vi "Init Stream.vi"(0 "Target IPAddress":string) -> ()   [LabVIEW 2015]
panel:
  out "Tab Control":enum32{"ON", "Off"}(tab)
  in  "Start":bool
  # "Start"
  # "Hi!\nThere are a few settings you will have to configure for the robot to run..."
  # "Please wait. Loading..."
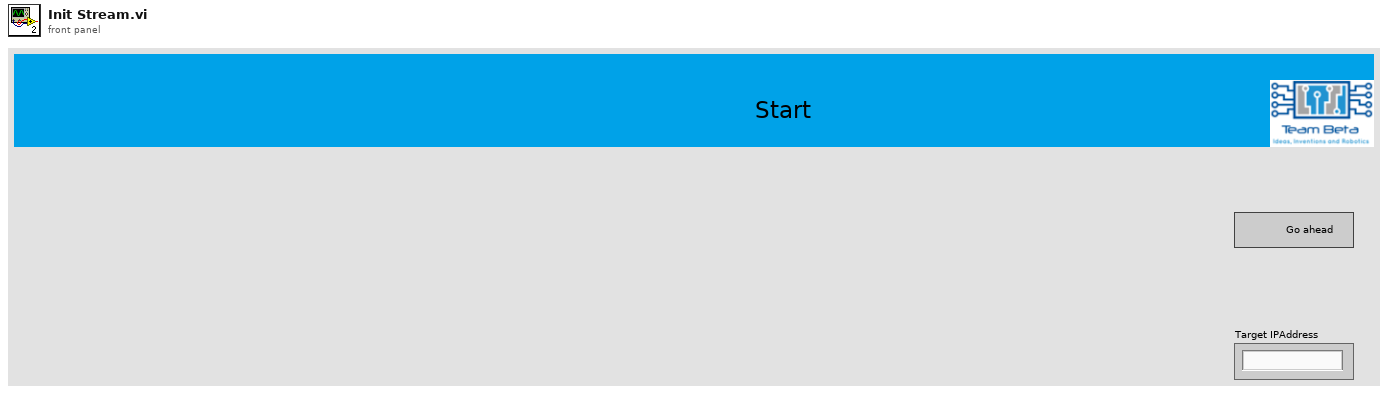
[diagram p1: front panel]
types:
  T1 = typedef "MODE.ctl" = enum8{"Protected Manaul", "Automatic", "Manaul"}
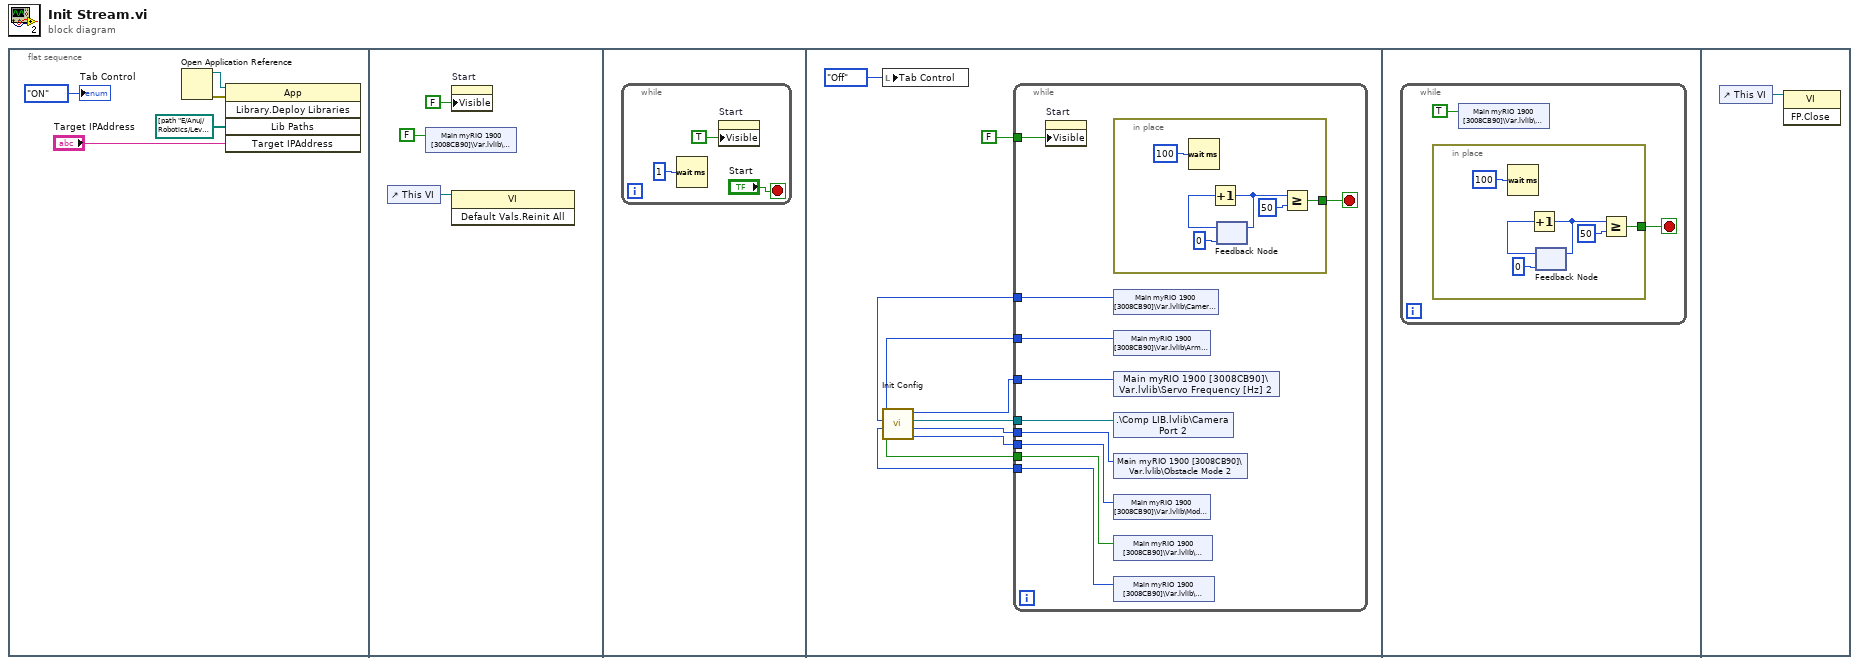
[diagram p0: block diagram]
diagram:
  n1 = flat-sequence {
    frame #0 {
      n2 = Open Application Reference() -> (0:w4:errorcluster, 3:w3:refnum<vi>)  [unwired: 4 in]
      n3 = invoke class="App" method="Library.Deploy Libraries"(reference=w3, error in=w4, "Lib Paths"=path[] [path "E:/Anuj/Robotics/Level 3/LabVIEW/Main VIs/LV15/PDMS/Real Time/Var.lvlib"] ("Library Paths"), "Target IPAddress"="Target IPAddress") -> ()  [unwired: 1 in, 5 out]
      "Tab Control" <- enum32{"ON", "Off"}."ON" ("Tab Control")
    }
    frame #1 {
      n4 = control-ref of="This VI"() -> (w8:refnum<vi>)
      n5 = shared-variable "Main myRIO 1900 [3008CB90]\\Var.lvlib\\Start-init"(FALSE ("Stop-init")) -> ()  [unwired: 1 in, 1 out]
      n6 = property on="Start" class="Bool"("Visible"=FALSE) -> ()  [unwired: 2 in, 2 out]
      n7 = invoke class="VI" method="Default Vals.Reinit All"(reference=w8) -> ()  [unwired: 2 in, 3 out]
    }
    frame #2 {
      n8 = while {
        stop <- "Start" stop-if-true
        n9 = Wait (ms)(milliseconds to wait=u32 1 ("millisecond timer value")) -> ()  [unwired: 1 out]
        n10 = property on="Start" class="Bool"("Visible"=TRUE) -> ()  [unwired: 2 in, 2 out]
      }
    }
    frame #3 {
      n11 = local write "Tab Control"(enum32{"ON", "Off"}."Off" ("Tab Control")) -> ()
      n12 = call "Init Config.vi"() -> ("Mode out"=w18:T1, "Obstacle Mode 2"=w19:u16, "Camera Port 2"=w15:refnum<k21>, "Servo Frequency [Hz] 2"=w20:u32, "Canceled?"=w17:bool, "Obstacle??"=w14:enum32{"Radio Selection 1", "Radio Selection 2"}, "Camera YN"=w13:enum32{"Radio Selection 1", "Radio Selection 2"}, "Arm Type"=w16:enum32{"RS1", "RS2"})  [unwired: 4 in]
      n13 = while {
        tunnel: FALSE ("Visible") -> [w30]
        tunnel: w20 -> [w29]
        tunnel: w19 -> [w28]
        tunnel: w18 -> [w27]
        tunnel: w17 -> [w26]
        tunnel: w16 -> [w25]
        tunnel: w15 -> [w24]
        tunnel: w14 -> [w23]
        tunnel: w13 -> [w22]
        stop <- w31 stop-if-true
        n14 = property on="Start" class="Bool"("Visible"=w30) -> ()  [unwired: 2 in, 2 out]
        n15 = in-place {
          in-place-border: [w32] -> w31
          n16 = Wait (ms)(milliseconds to wait=u32 100 ("millisecond timer value")) -> ()  [unwired: 1 out]
          n17 = feedback #1(u16 0) -> (w37:u16)
          n18 = Increment(x=w37) -> (x+1=w35:u16)
          n19 = feedback-in #1(w35) -> ()
          n20 = Greater Or Equal?(x=w35, y=u16 50) -> (x >= y?=w32:bool)
        }
        n21 = shared-variable "Main myRIO 1900 [3008CB90]\\Var.lvlib\\Camera YN"(w22) -> ()  [unwired: 1 in, 1 out]
        n22 = shared-variable "Main myRIO 1900 [3008CB90]\\Var.lvlib\\Arm Type"(w25) -> ()  [unwired: 1 in, 1 out]
        n23 = shared-variable "Main myRIO 1900 [3008CB90]\\Var.lvlib\\Servo Frequency [Hz] 2"(w29) -> ()  [unwired: 1 in, 1 out]
        n24 = shared-variable ".\\Comp LIB.lvlib\\Camera Port 2"(w24) -> ()  [unwired: 1 in, 1 out]
        n25 = shared-variable "Main myRIO 1900 [3008CB90]\\Var.lvlib\\Obstacle Mode 2"(w28) -> ()  [unwired: 1 in, 1 out]
        n26 = shared-variable "Main myRIO 1900 [3008CB90]\\Var.lvlib\\Mode out"(w27) -> ()  [unwired: 1 in, 1 out]
        n27 = shared-variable "Main myRIO 1900 [3008CB90]\\Var.lvlib\\Canceled?"(w26) -> ()  [unwired: 1 in, 1 out]
        n28 = shared-variable "Main myRIO 1900 [3008CB90]\\Var.lvlib\\Obstacle??"(w23) -> ()  [unwired: 1 in, 1 out]
      }
    }
    frame #4 {
      n29 = while {
        stop <- w38 stop-if-true
        n30 = in-place {
          in-place-border: [w40] -> w38
          n31 = Wait (ms)(milliseconds to wait=u32 100 ("millisecond timer value")) -> ()  [unwired: 1 out]
          n32 = feedback #2(u16 0) -> (w45:u16)
          n33 = Increment(x=w45) -> (x+1=w43:u16)
          n34 = feedback-in #2(w43) -> ()
          n35 = Greater Or Equal?(x=w43, y=u16 50) -> (x >= y?=w40:bool)
        }
        n36 = shared-variable "Main myRIO 1900 [3008CB90]\\Var.lvlib\\Start-init"(TRUE) -> ()  [unwired: 1 in, 1 out]
      }
    }
    frame #5 {
      n37 = control-ref of="This VI"() -> (w46:refnum<vi>)
      n38 = invoke class="VI" method="FP.Close"(reference=w46) -> ()  [unwired: 2 in, 3 out]
    }
  }
